vi "TipPokeQualityOfLife.vi"() -> ()   [LabVIEW 2021]
uses:
  <userlib>/Nanonis Prog Interface V5/Nanonis Prog Interface.lvlib
panel:
  in  "Shape TipLift (m)":dbl=-1.3e-09 format="%#_6p"
  in  "Shape lifting bias (V)":dbl=2.0
  in  "Spectrum TipLift (m)":dbl=-1e-09 format="%#_6p"
  in  "Spectrum lifting bias (V)":dbl=-1.0
  in  "Shape poke":bool
  in  "Spectrum poke":bool
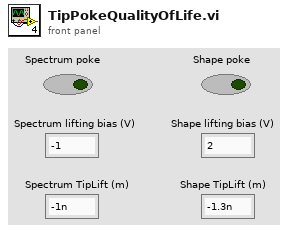
[diagram p1: front panel]
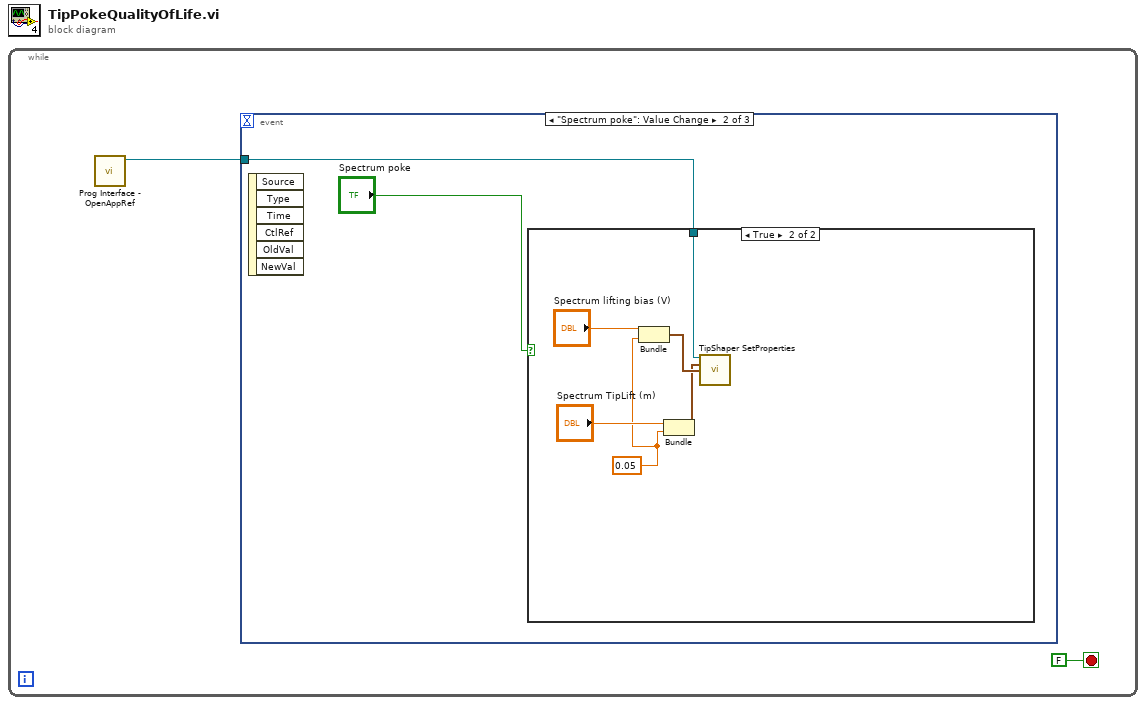
[diagram p0: block diagram]
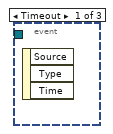
[diagram p2: hidden frame]
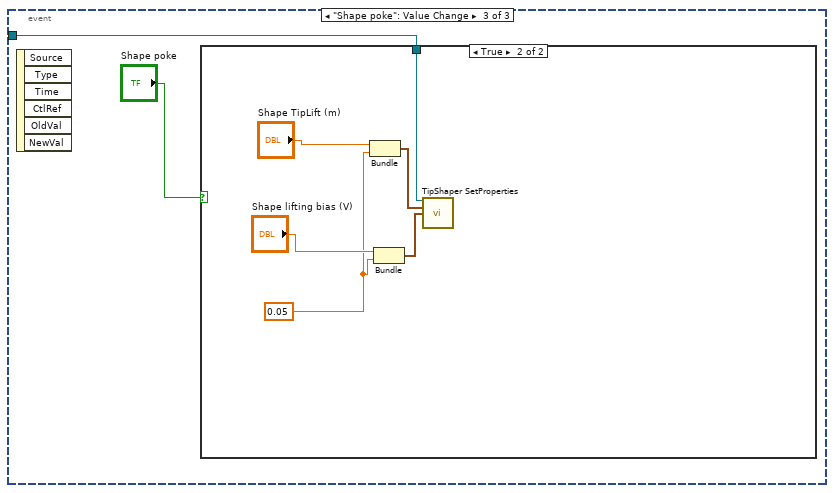
[diagram p4: hidden frame]
diagram:
  n1 = while {
    stop <- FALSE stop-if-true
    n2 = call <userlib>:"Prog Interface - OpenAppRef.vi"() -> ("Application reference"=w2:refnum<vi>)  [unwired: 6 in, 1 out]
    n3 = event shown="[1] \"Spectrum poke\": Value Change" {
      selector: _ -> [_ _ _]
      dyn-events: _ -> [_ _ _]
      timeout: _ -> [_ _ _]
      tunnel: w2 -> [_ w3 w11]
      event Timeout {
        n4 = event-data() -> ()  [unwired: 1 in, 3 out]
      }
      event "Spectrum poke": Value Change {
        n5 = event-data() -> ()  [unwired: 1 in, 6 out]
        n6 = case shown="True" "Spectrum poke" {
          tunnel: w3 -> [_ w10]
          frame False {
          }
          frame True {
            w7 = 0.05
            n7 = Bundle("Spectrum lifting bias (V)"="Spectrum lifting bias (V)", w7) -> (w6:cluster{"Spectrum lifting bias (V)":dbl, dbl})  [unwired: 1 in]
            n8 = Bundle("Spectrum TipLift (m)"="Spectrum TipLift (m)", w7) -> (w5:cluster{"Spectrum TipLift (m)":dbl, dbl})  [unwired: 1 in]
            n9 = call <userlib>:"TipShaper SetProperties.vi"("Application ref in"=w10, "Tip Lift 1"=w5, "Bias Lift"=w6) -> ()  [unwired: 11 in, 2 out]
          }
        }
      }
      event "Shape poke": Value Change {
        n10 = event-data() -> ()  [unwired: 1 in, 6 out]
        n11 = case shown="True" "Shape poke" {
          tunnel: w11 -> [_ w18]
          frame False {
          }
          frame True {
            w14 = 0.05
            n12 = Bundle("Shape TipLift (m)"="Shape TipLift (m)", w14) -> (w16:cluster{"Shape TipLift (m)":dbl, dbl})  [unwired: 1 in]
            n13 = Bundle("Shape lifting bias (V)"="Shape lifting bias (V)", w14) -> (w13:cluster{"Shape lifting bias (V)":dbl, dbl})  [unwired: 1 in]
            n14 = call <userlib>:"TipShaper SetProperties.vi"("Application ref in"=w18, "Tip Lift 1"=w16, "Bias Lift"=w13) -> ()  [unwired: 11 in, 2 out]
          }
        }
      }
    }
  }
